vi "SENS_IF_FILT_STAGE_COUN.vi"(0 "VISA IN":refnum<visa-resource-name>, 1 "Stage number":i32, 2 "Optional Parameter":string, 5 "error in":errorcluster, 7 "Channel":i32) -> (14 "VISA Out":refnum<visa-resource-name>, 16 "Data":string, 19 "error out":errorcluster)   [LabVIEW 2018, in "PNA-X.lvlib"]
doc: "SENSe<cnum>:IF:FILTer:STAGE<n>:COUNt? [char] \n(Read-only) Returns the number of taps in the digital filter of the specified stage. The filter sample \ncount setting is only used when SENSe:IF:FILTer:AUTO is set to False (MANUAL). \nCritical Note \nParameters \n<cnum> Existing channel number. If unspecified, <cnum> is set to 1. \n<n> Stage number. Choose 1 or 2 \n[char] Optional parameter. Choose from: \nnot specified - returns the current number of coefficients for the specified \nstage. \nMIN - returns the minimum number of coefficients for the specified \nstage. Stage1: 10, Stage2: 1 \nMAX - returns the maximum number of coefficients for the specified \nstage. Stage1 & 2: 1024 \nExamples SENS:IF:FILT:STAG2:COUN? \nsense2:if:filter:stage1:count? max \nReturn Type Numeric \nDefault Stage dependent \n1756"
uses:
  PNA-X.lvlib
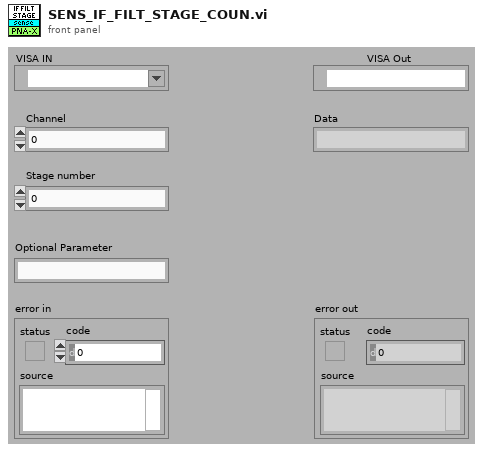
[diagram p1: front panel]
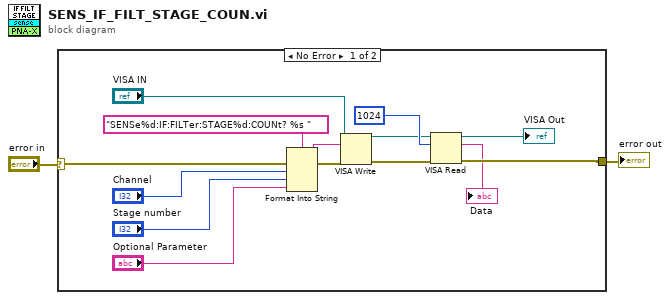
[diagram p0: block diagram]
diagram:
  n1 = case shown="No Error" "error in" {
    selector: "error in" -> [w16 w17]
    tunnel: [w7 w17] -> w1
    frame No Error {
      n2 = Format Into String(format string="SENSe%d:IF:FILTer:STAGE%d:COUNt? %s " ("Cmdline"), error in=w16, "Channel", "Stage number", "Optional Parameter") -> (resulting string=w14:string, error out=w15:errorcluster)  [unwired: 1 in]
      n3 = VISA Write(VISA resource name="VISA IN", write buffer=w14, error in (no error)=w15) -> (VISA resource name out=w9:refnum<visa-resource-name>, error out=w11:errorcluster)  [unwired: 1 out]
      n4 = VISA Read(VISA resource name=w9, byte count=1024, error in (no error)=w11) -> (VISA resource name out=→"VISA Out":refnum<visa-resource-name>, read buffer=→"Data":string, error out=w7:errorcluster)  [unwired: 1 out]
    }
    frame Error {
    }
  }
  "error out" <- w1
